vi "Calib IAS v0.1.vi"(7 "Mean Dimension":dbl format="%#_13g", 8 "x 4":dbl, 9 "x 3":dbl, 10 "x 2":dbl, 11 "x":dbl) -> (0 "y 4":dbl, 1 "y 3":dbl, 2 "y 2":dbl, 3 "y 1":dbl, 4 "Output Parts":T1, 5 "Auto":dbl[](array[numeric]))   [LabVIEW 2021]
uses:
  Global Variables/RT GV.vi
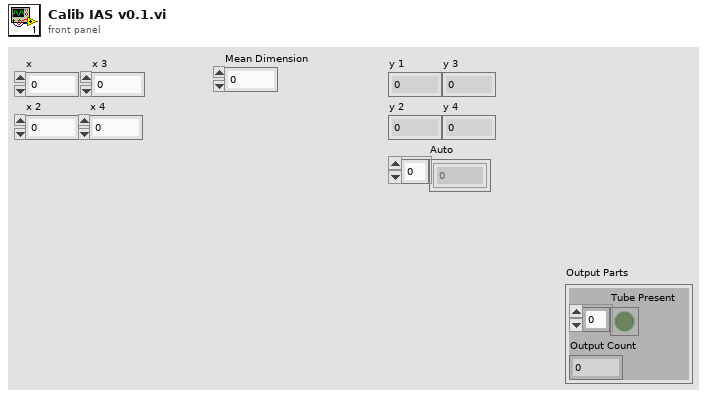
[diagram p1: front panel]
types:
  T1 = cluster{"Tube Present":bool[], "Output Count":u32}
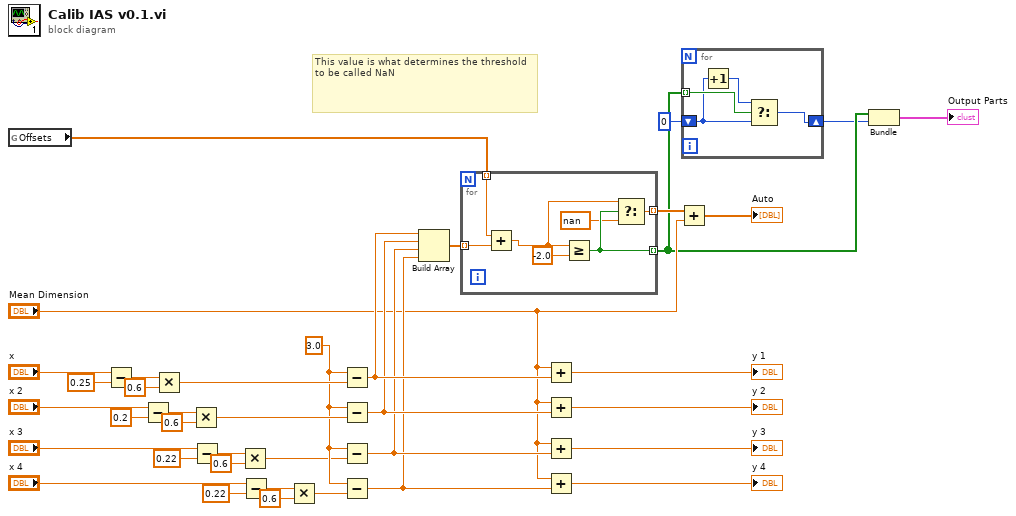
[diagram p0: block diagram]
diagram:
  w20 = 3.0 ("y")
  # "This value is what determines the threshold to be called NaN"
  n1 = global read "RT GV.vi" "Offsets"() -> (w1:dbl[])
  n2 = Subtract(x="x", y=0.25) -> (x-y=w37:dbl)
  n3 = Subtract(x="x 2", y=0.2) -> (x-y=w34:dbl)
  n4 = Multiply(x=w37, y=0.6) -> (x*y=w22:dbl)
  n5 = Multiply(x=w34, y=0.6) -> (x*y=w21:dbl)
  n6 = Subtract(x="x 3", y=0.22) -> (x-y=w31:dbl)
  n7 = Multiply(x=w31, y=0.6) -> (x*y=w19:dbl)
  n8 = Subtract(x="x 4", y=0.22) -> (x-y=w28:dbl)
  n9 = Multiply(x=w28, y=0.6) -> (x*y=w18:dbl)
  n10 = Subtract(x=w20, y=w22) -> (x-y=w13:dbl)
  n11 = Subtract(x=w20, y=w21) -> (x-y=w12:dbl)
  n12 = Subtract(x=w20, y=w19) -> (x-y=w11:dbl)
  n13 = Subtract(x=w20, y=w18) -> (x-y=w10:dbl)
  n14 = Build Array(w13, w12, w11, w10) -> (w9:dbl[])
  n15 = for {
    tunnel: w9 -> [w41] mode=indexing
    tunnel: [w44] -> w4 mode=indexing
    tunnel: [w43] -> w7 mode=indexing
    tunnel: w1 -> [w39] mode=indexing
    n16 = Add(x=w39, y=w41) -> (x+y=w40:dbl)
    n17 = Greater Or Equal?(x=w40, y=-2.0) -> (x >= y?=w44:bool)
    n18 = Select(t=w40, s=w44, f=nan) -> (s? t:f=w43:dbl)
  }
  n19 = Add(x="Mean Dimension", y=w13) -> (x+y=→"y 1":dbl)
  n20 = Add(x="Mean Dimension", y=w12) -> (x+y=→"y 2":dbl)
  n21 = Add(x="Mean Dimension", y=w11) -> (x+y=→"y 3":dbl)
  n22 = Add(x="Mean Dimension", y=w10) -> (x+y=→"y 4":dbl)
  n23 = Add(x=w7, y="Mean Dimension") -> (x+y=→"Auto":dbl[])
  n24 = for {
    tunnel: w4 -> [w49] mode=indexing
    shift-right: [w48] -> w3
    shift-left: u32 0 -> [w47]
    n25 = Increment(x=w47) -> (x+1=w46:u32)
    n26 = Select(t=w46, s=w49, f=w47) -> (s? t:f=w48:u32)
  }
  n27 = Bundle(w4, w3) -> (→"Output Parts":cluster{bool[], u32})  [unwired: 1 in]
